vi "KE622x -- Set Voltage Limit.vi"(0 "Resource In":refnum<visa-resource-name>, 1 "Check For SCPI Errors? (T)":bool=TRUE, 7 "Voltage Limit (V)":T1=10.0 min=0.1 max=105.0 step=0.01 format="%.2p", 11 "error in (no error)":errorcluster) -> (4 "Resource Out (dupl)":refnum<visa-resource-name>, 15 "error out":errorcluster)   [LabVIEW 2013, in "Keithly user program.lvlib"]
doc: "Sets the voltage limit (compliance) for the current source."
uses:
  Keithly user program.lvlib
  Typedefs/KE622x -- Voltage Limit.ctl
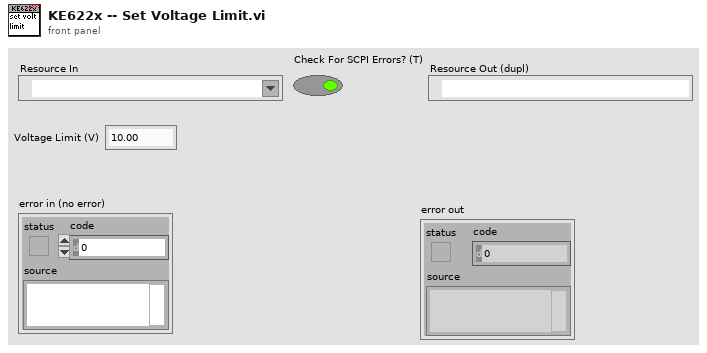
[diagram p1: front panel]
types:
  T1 = typedef "Keithly user program.lvlib/KE622x -- Voltage Limit.ctl" = dbl
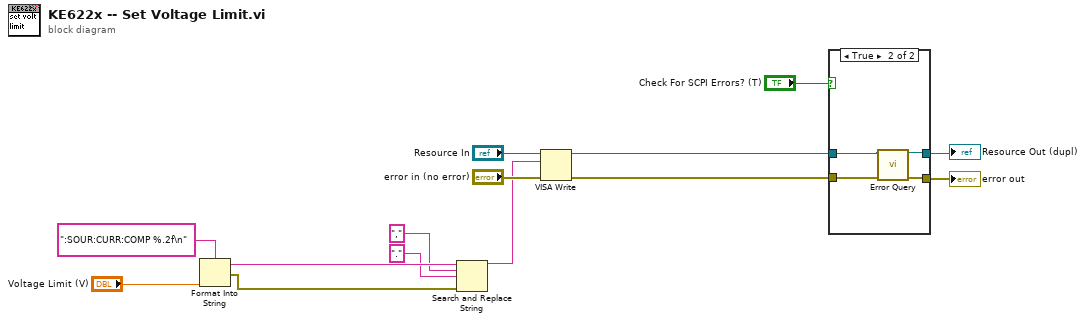
[diagram p0: block diagram]
diagram:
  n1 = Format Into String(format string=":SOUR:CURR:COMP %.2f\n", "Voltage Limit (V)") -> (resulting string=w6:string, error out=w5:errorcluster)  [unwired: 2 in]
  n2 = Search and Replace String(input string=w6, search string=",", replace string="." ("replace string (\"\")"), error in=w5) -> (result string=w4:string)  [unwired: 4 in, 3 out]
  n3 = VISA Write(VISA resource name="Resource In", write buffer=w4, error in (no error)="error in (no error)") -> (VISA resource name out=w10:refnum<visa-resource-name>, error out=w9:errorcluster)  [unwired: 1 out]
  n4 = case shown="True" "Check For SCPI Errors? (T)" {
    tunnel: w10 -> [w16 w20]
    tunnel: w9 -> [w15 w18]
    tunnel: [w15 w17] -> w7
    tunnel: [w16 w19] -> w8
    frame False {
    }
    frame True {
      n5 = call "Error Query.vi"("VISA Resource In"=w20, "error in (no error)"=w18) -> ("VISA Resource Out (dupl)"=w19:refnum<visa-resource-name>, "error out"=w17:errorcluster)  [unwired: 10 in, 2 out]
    }
  }
  "Resource Out (dupl)" <- w8
  "error out" <- w7
